vi "Update Armed.vi"(8 "error in (no error)":errorcluster, 10 "Armed":bool, 11 "Monitor-Pulse in":refnum<class "Monitor-Pulse.lvclass">) -> (0 "error out":errorcluster, 3 "Monitor-Pulse out":refnum<class "Monitor-Pulse.lvclass">)   [LabVIEW 2015, in "Monitor-Pulse.lvclass"]
uses:
  Monitor-Pulse.lvclass
  Monitor-Pulse.lvclass/Monitor-Pulse.ctl
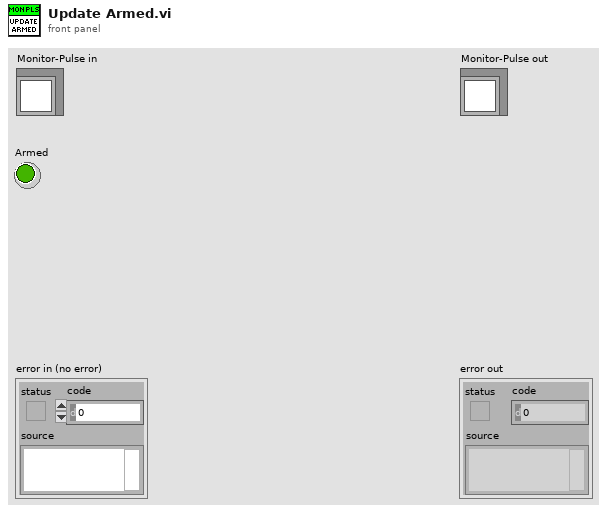
[diagram p1: front panel]
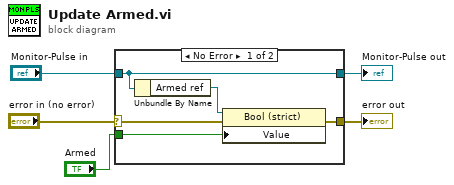
[diagram p0: block diagram]
diagram:
  n1 = case shown="No Error" "error in (no error)" {
    selector: "error in (no error)" -> [w7 w12]
    tunnel: [w6 w12] -> w4
    tunnel: [w10 w11] -> w2
    tunnel: "Monitor-Pulse in" -> [w10 w11]
    tunnel: "Armed" -> [w8 _]
    frame No Error {
      n2 = Unbundle By Name(w10) -> ("Armed ref"=w9:refnum<vi>)
      n3 = property class="Bool (strict)"(reference=w9, error in=w7, "Value"=w8) -> (error out=w6:errorcluster)  [unwired: 1 out]
    }
    frame Error {
    }
  }
  "error out" <- w4
  "Monitor-Pulse out" <- w2
